vi "Simple_ManualSyringeControl_VB_20170921_synchronousflush.vi"() -> ()   [LabVIEW 2013]
uses:
  <vilib>/Instr/_visa.llb/VISA Configure Serial Port (Instr).vi
  <vilib>/Instr/_visa.llb/VISA Flush IO Buffer Mask.ctl
panel:
  out "Syringe Diameter (mm)":string
  in  "Mask":T1=16 items=["Flush Receive Buffer"=16, "Write Transmit Buffer to Device"=32, "Flush Receive Buffer (No I/O)"=64, "Flush Transmit Buffer"=128]
  out "Pump #":dbl caption="Pumps:" format="%#g"
  out "Sync":bool
  in  "STOP ALL":bool
  in  "RUN ALL":bool
  in  "Synchronous Pumps (T/F)":bool
  in  "Flush Rate (mL/hour)":string="20"
  out "Flushing?":bool
  in  "Flush":bool
  in  "Infuse Rate (mL/hour)":string="2"
  in  "STOP PUMP 01":bool
  in  "RUN PUMP 01":bool
  in  "Mask Init 2":T1=16 items=["Flush Receive Buffer"=16, "Write Transmit Buffer to Device"=32, "Flush Receive Buffer (No I/O)"=64, "Flush Transmit Buffer"=128]
  in  "stop bits (2 bit)":u16(ring)=20 items=["1.0"=10, "1.5"=15, "2.0"=20]
  in  "termination char\n(0xD = '\\r' = CR)":u8=13 format="%.0x"
  in  "data bits (8)":u16=8 min=5 max=8 step=1
  in  "baud rate (9600)":u32=9600
  in  "VISA resource name":refnum<visa-resource-name>="COM3"
  in  "STOP PUMP 00":bool
  in  "Mask Exit":T1=16 items=["Flush Receive Buffer"=16, "Write Transmit Buffer to Device"=32, "Flush Receive Buffer (No I/O)"=64, "Flush Transmit Buffer"=128]
  in  "RUN PUMP 00":bool
  in  "Mask Initialize 2":T1=16 items=["Flush Receive Buffer"=16, "Write Transmit Buffer to Device"=32, "Flush Receive Buffer (No I/O)"=64, "Flush Transmit Buffer"=128]
  in  "Mask Init":T1=16 items=["Flush Receive Buffer"=16, "Write Transmit Buffer to Device"=32, "Flush Receive Buffer (No I/O)"=64, "Flush Transmit Buffer"=128]
  out "Response":string
  out "Response Blank":string
  in  "Command:":string
  in  "Pump Address":enum16{"00", "01", "02", "03"}(ring)
  in  "OK Button":bool
  in  "EXIT PROGRAM":bool
  # "UPON START-UP: User is asked to input number of pumps being used and diameter of syringe"
  # "DURING RUN: Default Infusion Rate is 2 mL/hour, to change this, modify Infusion Rate before giving RUN command or pressing PLAY"
  # "OFF"
  # "ON"
  # "COMMANDS LIST\n\nRUN Start infuse (forward direction)\nRUNW Starts withdraw (reverse direction)\nSTP Stop motor\nCLV Clears infuse volume accumulator to zero\nCLT Clears target infuse volume to zero, dispense disabled\nCLTW Clears target withdraw volume to zero\nMAX Sets the pump to the maximum infuse flow rate\n\nCommands with Numbers \n(Number Range: 0-1999)\n(Must have space before number)\nFOR Force setting as percentage (number can be 0-100).\nMLH Set infuse flow rate and range, units are milliliters per hour.\nULT  Set target infusion volume, units are µl .\nMLT Set target infusion volume, units are ml.\n\nSee Harvard Apparatus OEM Millimeter pump manual for more commands and details."
  # "QUERIES LIST \n\nDIA Returns diameter value units in mm\nRAT Returns infusion rate value set in current range units\nRATW Returns withdraw rate value set in current range units\nVOL Returns current accumulated infused volume, units in ml or µl\ndepending on range.\nVOLW Returns current accumulated withdraw volume, units in ml or µl\ndepending on range.\nVER Returns model and version number of firmware\nTAR Returns target infuse volume, units in ml or µl depending on range \nFRC Returns force setting and percent\nRNG Returns infuse range message (character string either: ML/H, ML/M,\nUL/H, UL/M)\nEMG Returns emergency stop input status (True/False); True =\nEmergency Stop\nLIM Returns “*I”, “*W” or “false”; indicating limit switch actuation status."
  # "Individual Control"
  # ": stopped\n> running forward\n*I stalled"
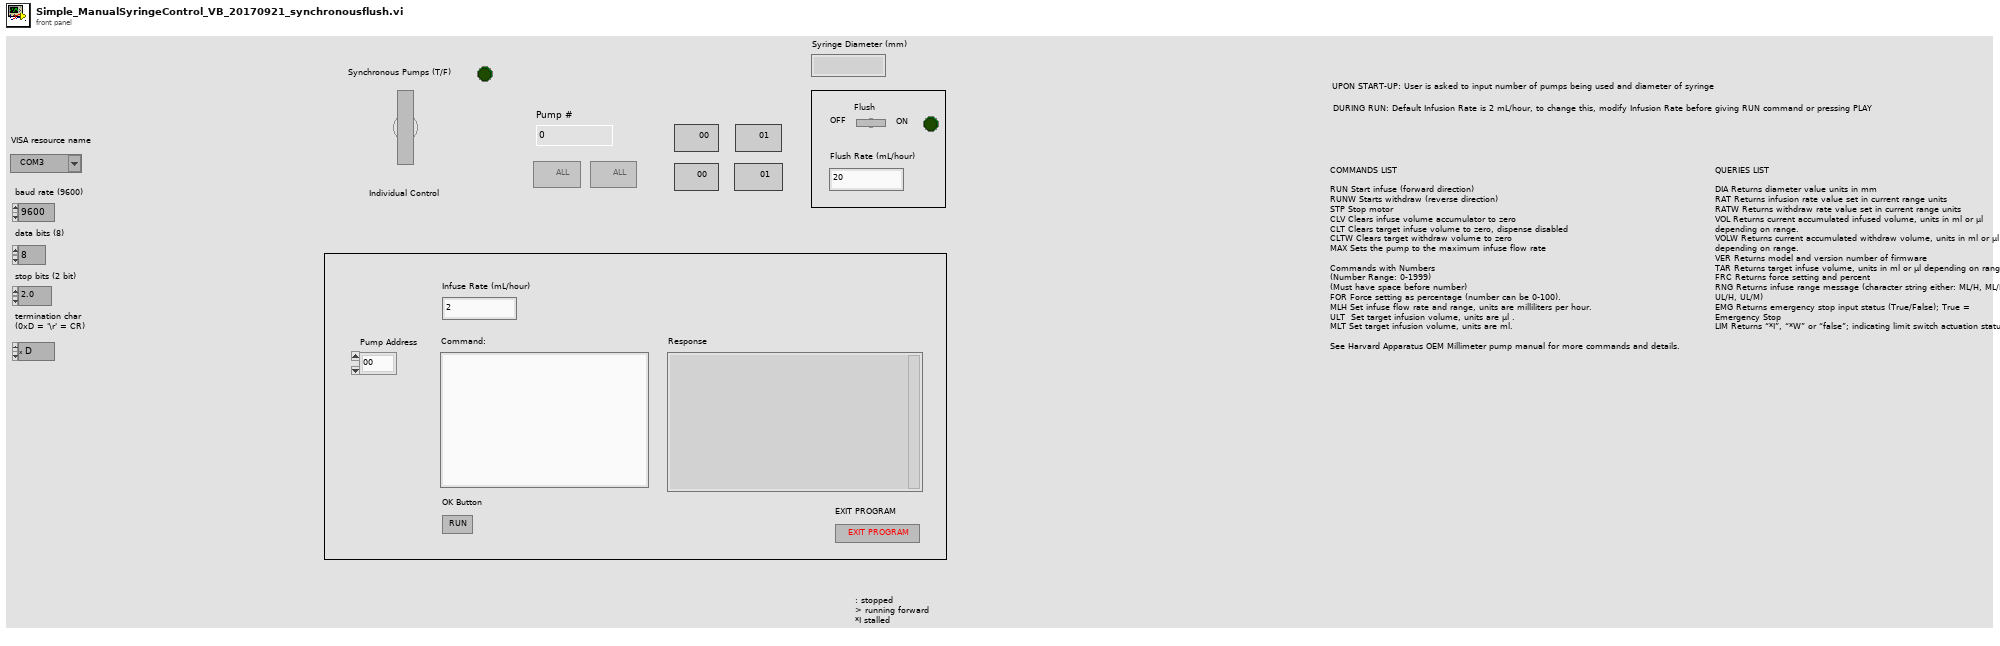
[diagram p1: front panel]
types:
  T1 = typedef "VISA Flush IO Buffer Mask.ctl" = u16
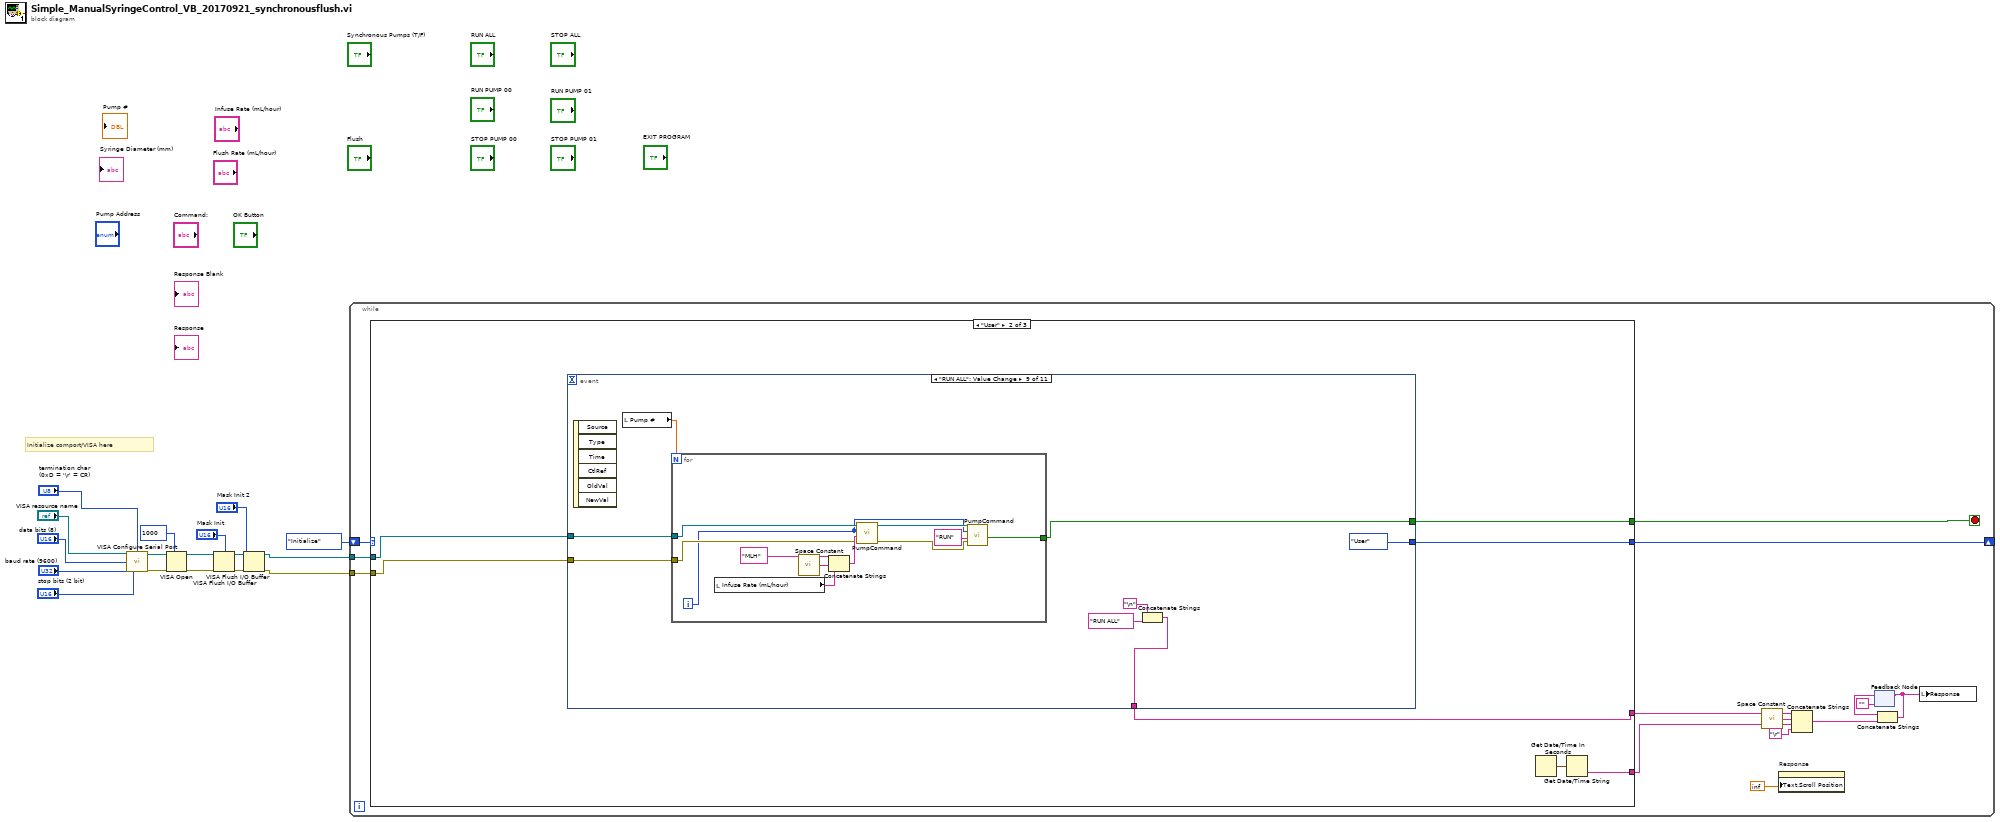
[diagram p0: block diagram]
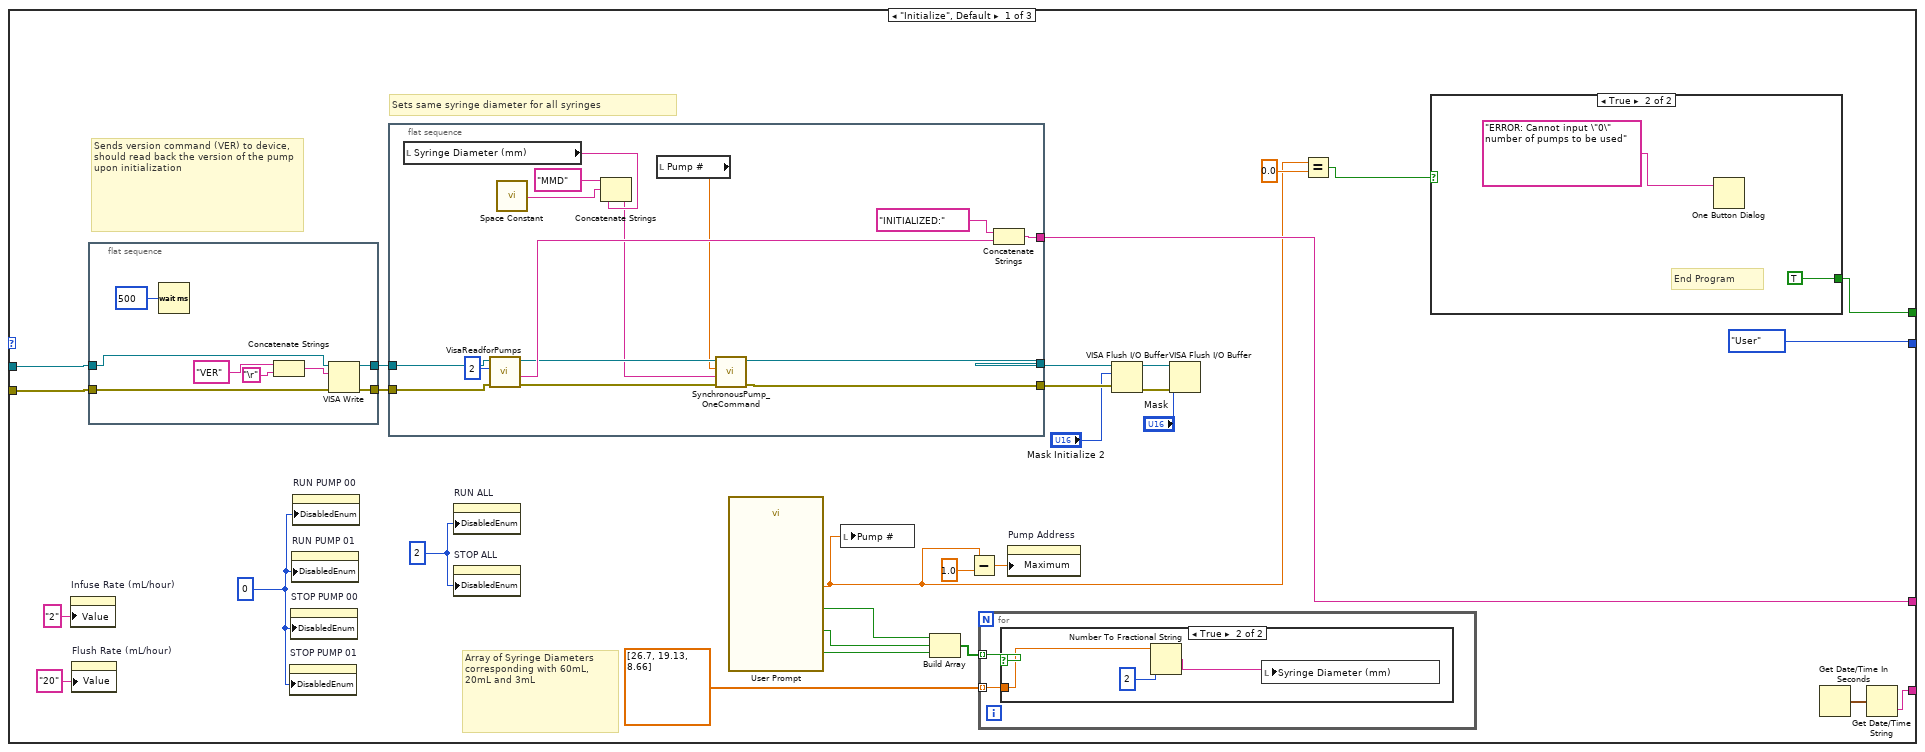
[diagram p2: hidden frame]
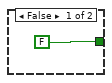
[diagram p3: hidden frame]
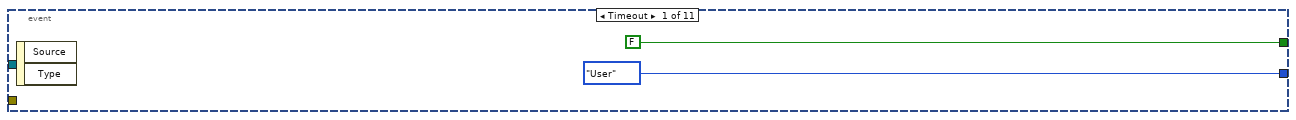
[diagram p5: hidden frame]
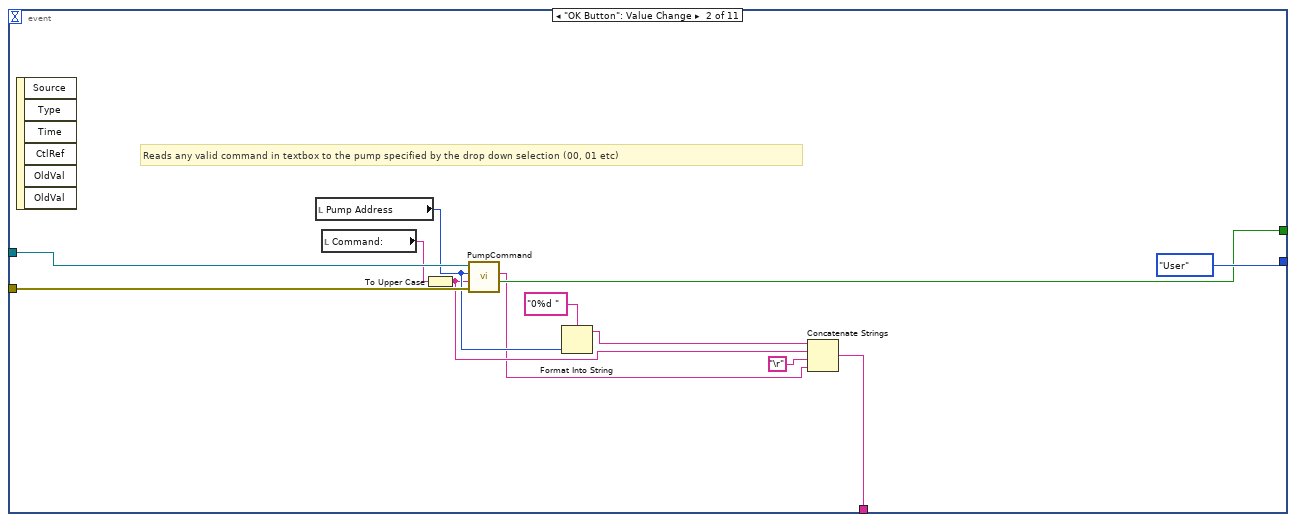
[diagram p6: hidden frame]
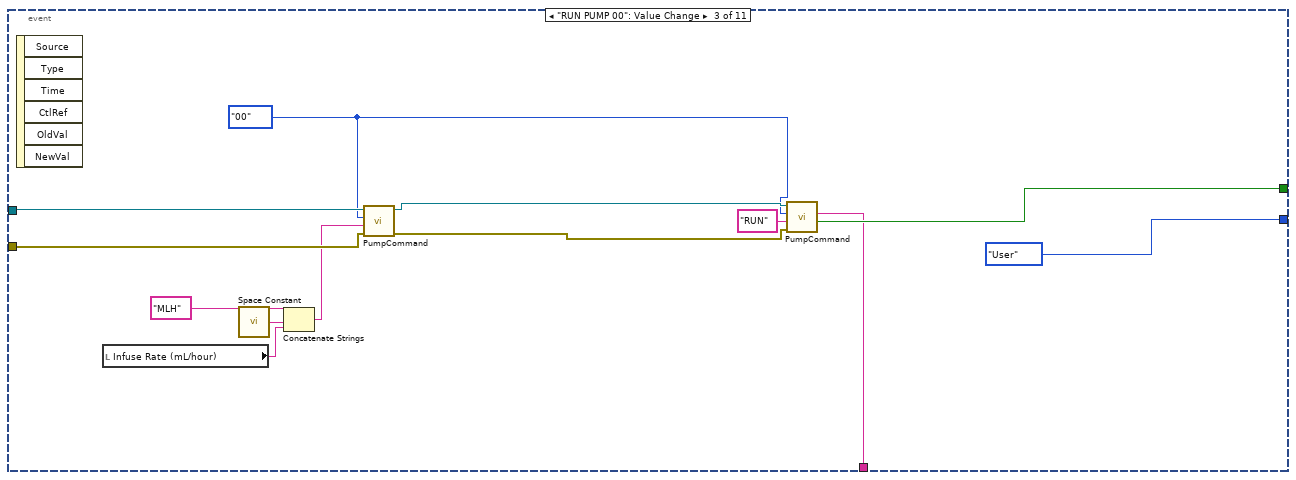
[diagram p7: hidden frame]
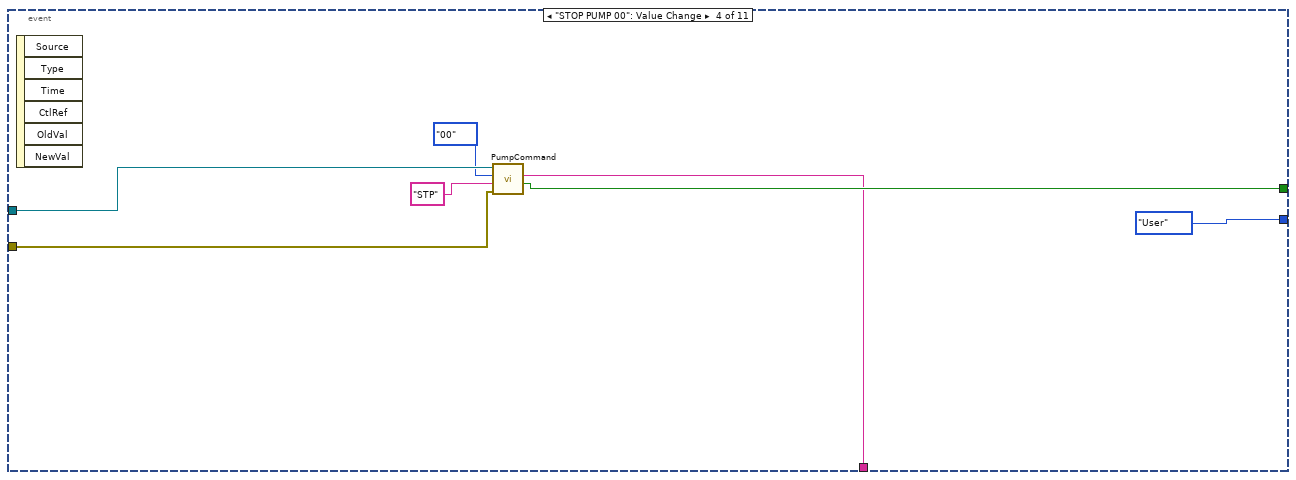
[diagram p8: hidden frame]
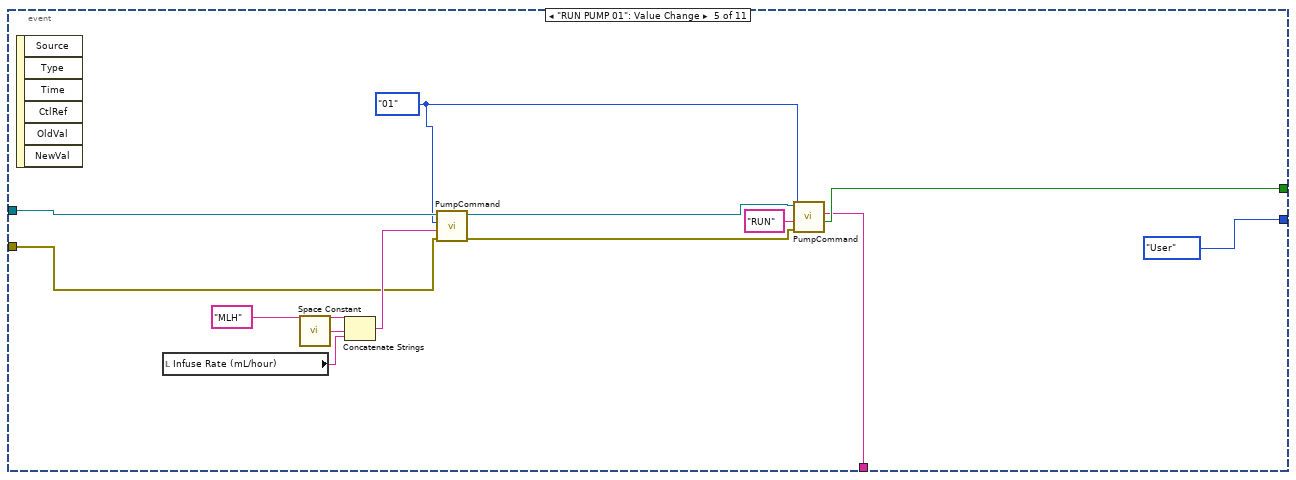
[diagram p9: hidden frame]
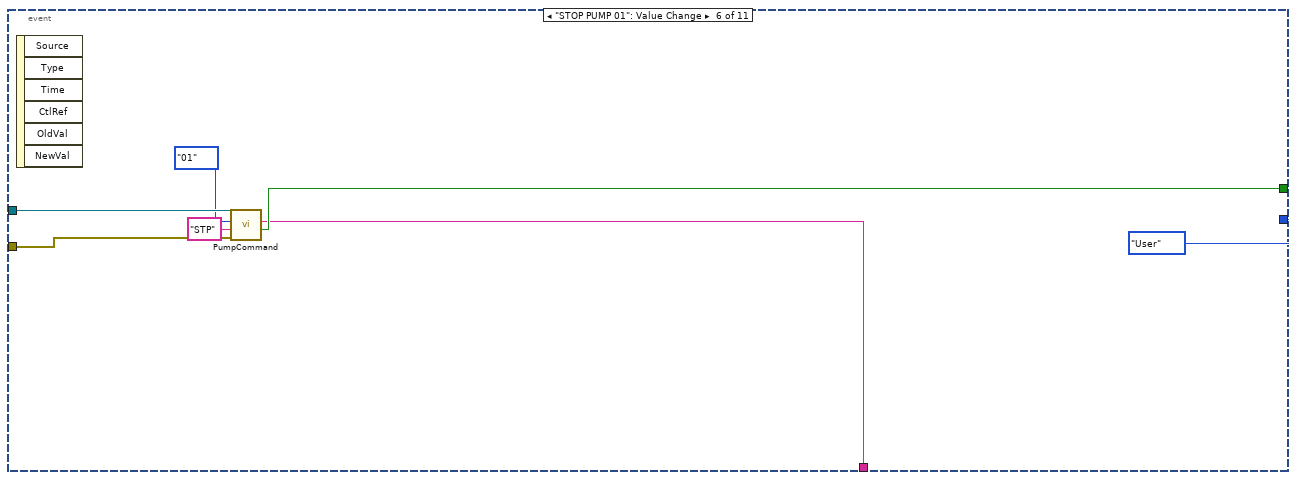
[diagram p10: hidden frame]
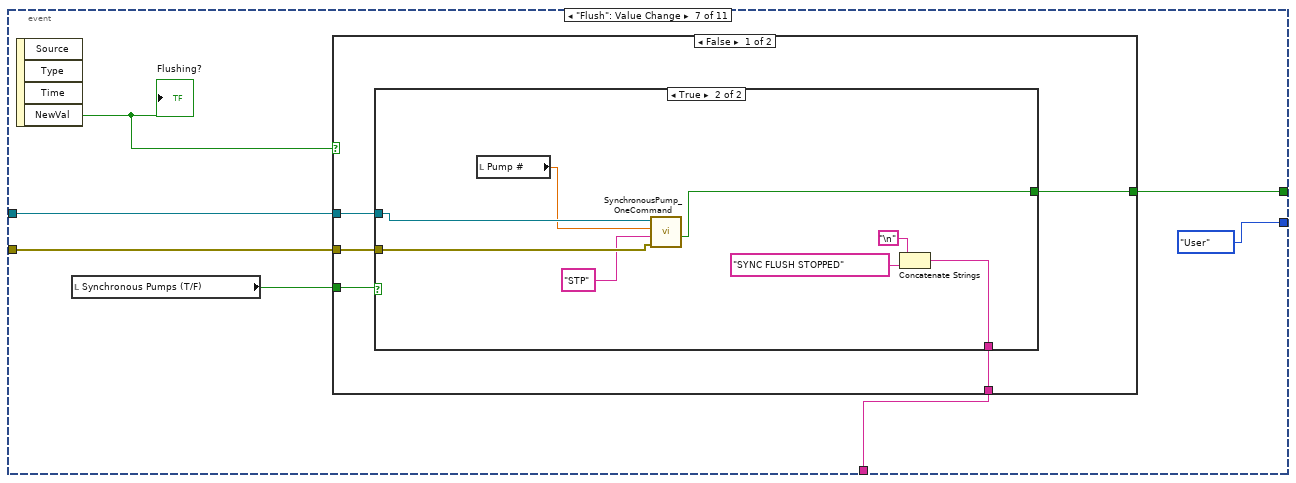
[diagram p11: hidden frame]
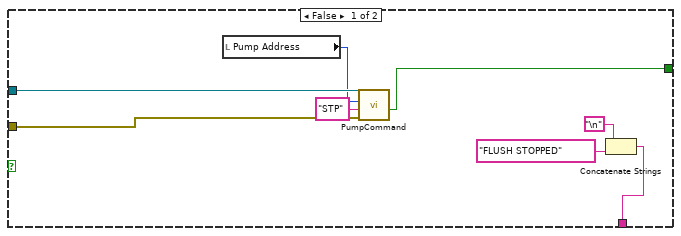
[diagram p12: hidden frame]
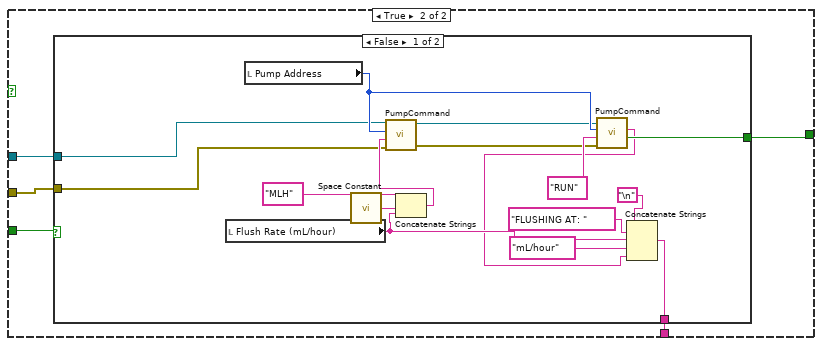
[diagram p13: hidden frame]
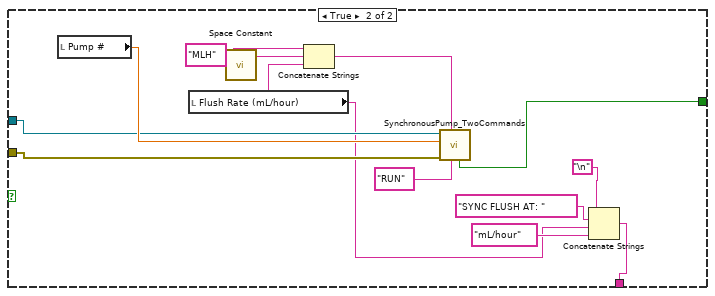
[diagram p14: hidden frame]
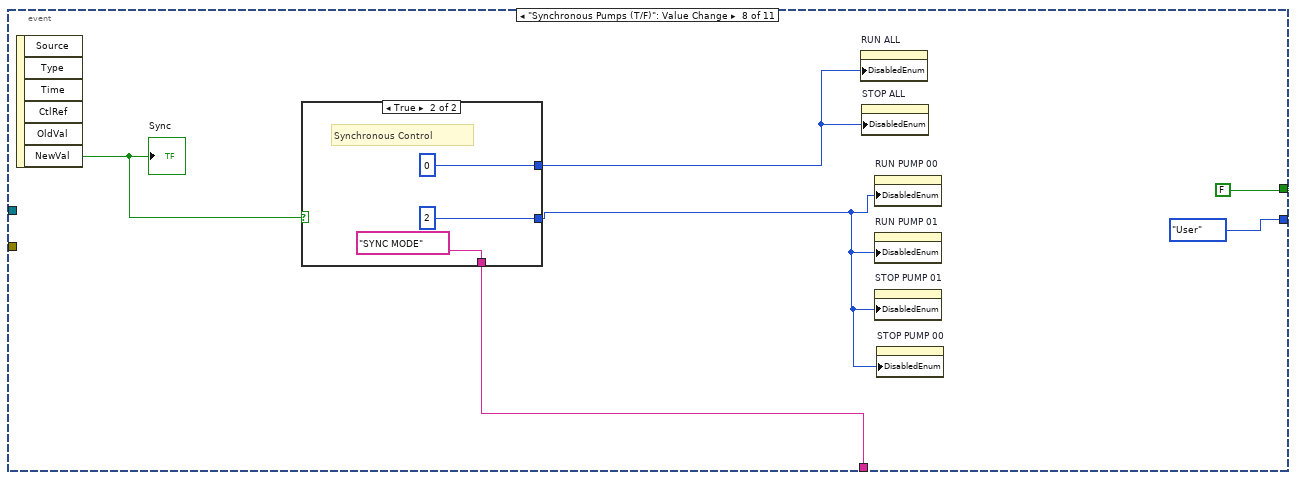
[diagram p15: hidden frame]
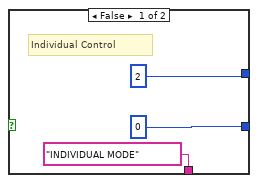
[diagram p16: hidden frame]
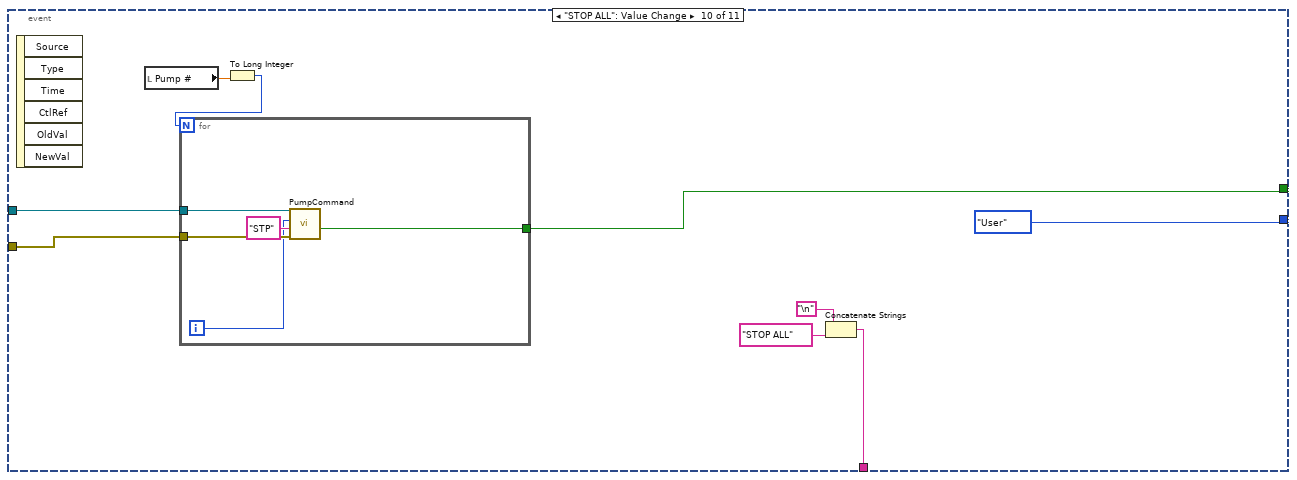
[diagram p17: hidden frame]
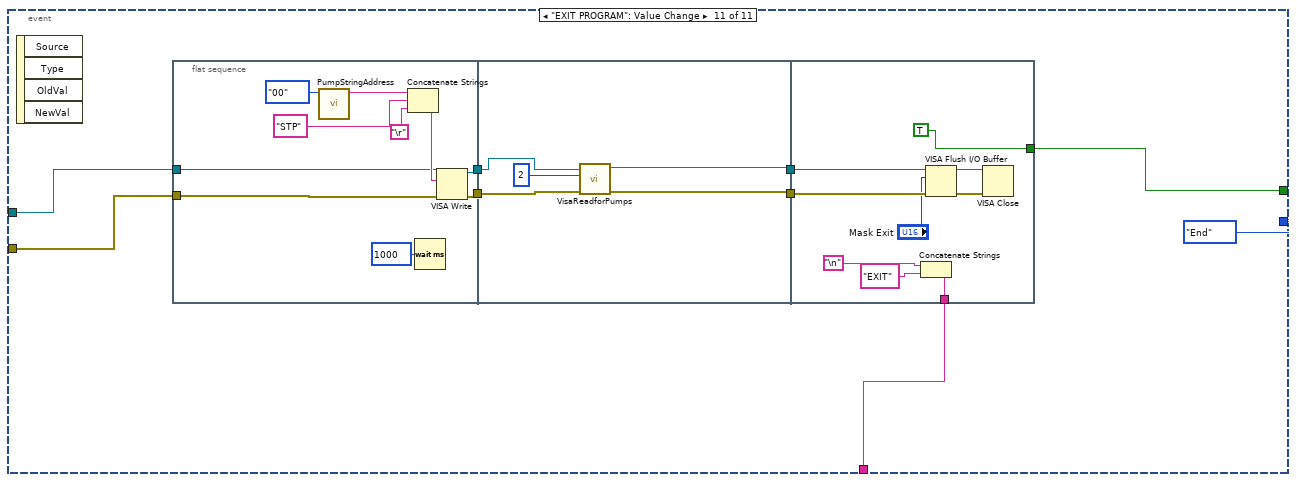
[diagram p18: hidden frame]
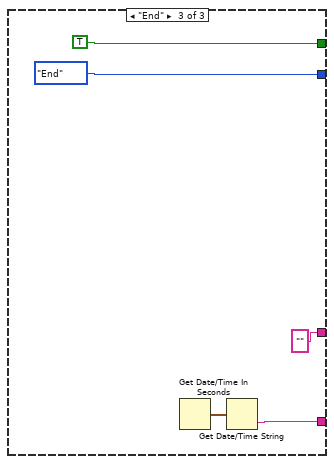
[diagram p19: hidden frame]
diagram:
  # "Initialize comport/VISA here"
  n1 = call-poly "VISA Configure Serial Port"("VISA resource name"="VISA resource name", "termination char\n(0xA = '\\n' = LF)"="termination char\n(0xD = '\\r' = CR)", "baud rate (9600)"="baud rate (9600)", "data bits (8)"="data bits (8)", "stop bits (10: 1 bit)"="stop bits (2 bit)") -> ("VISA resource name out"=w13:refnum<visa-resource-name>, "error out"=w12:errorcluster)  [unwired: 9 in]
  n2 = VISA Open(timeout (0)=1000, error in (no error)=w12, VISA resource name=w13) -> (VISA resource name=w15:refnum<visa-resource-name>, error out=w16:errorcluster)  [unwired: 2 in]
  n3 = VISA Flush I/O Buffer(VISA resource name=w15, mask (16)="Mask Init", error in (no error)=w16) -> (VISA resource name out=w4:refnum<visa-resource-name>, error out=w5:errorcluster)
  n4 = VISA Flush I/O Buffer(VISA resource name=w4, mask (16)="Mask Init 2", error in (no error)=w5) -> (VISA resource name out=w3:refnum<visa-resource-name>, error out=w2:errorcluster)
  n5 = while {
    shift-right: [w30] -> _
    shift-left: enum16{"Initialize", "User", "End"}."Initialize" -> [w29]
    tunnel: w3 -> [w28]
    tunnel: w2 -> [w27]
    stop <- w31 stop-if-true
    n6 = case shown="\"User\"" w29 {
      tunnel: [w33 w97 TRUE] -> w31
      tunnel: [enum16{"Initialize", "User", "End"}."User" w98 enum16{"Initialize", "User", "End"}."End"] -> w30
      tunnel: w28 -> [w55 w96 _]
      tunnel: w27 -> [w54 w95 _]
      tunnel: [w48 w94 "" ("Read (Response)")] -> w21
      tunnel: [w36 w92 w293] -> w18
      frame "Initialize", Default {
        w51 = 2
        w52 = 0
        # "Array of Syringe Diameters corresponding with 60mL, 20mL and 3mL"
        # "Sets same syringe diameter for all syringes"
        # "Sends version command (VER) to device, should read back the version of the pump upon initialization"
        n7 = property on="Infuse Rate (mL/hour)" class="Str"("Value"="2" ("Infuse Rate (mL/hour)")) -> ()  [unwired: 2 in, 2 out]
        n8 = property on="Flush Rate (mL/hour)" class="Str"("Value"="20" ("Flush Rate (mL/hour)")) -> ()  [unwired: 2 in, 2 out]
        n9 = flat-sequence {
          tunnel: [w89] -> w60
          tunnel: [w88] -> w59
          tunnel: w55 -> [w86]
          tunnel: w54 -> [w85]
          frame #0 {
            n10 = Wait (ms)(milliseconds to wait=500) -> ()  [unwired: 1 out]
            n11 = Concatenate Strings("VER", "\r") -> (w90:string)
            n12 = VISA Write(VISA resource name=w86, write buffer=w90, error in (no error)=w85) -> (VISA resource name out=w89:refnum<visa-resource-name>, error out=w88:errorcluster)  [unwired: 1 out]
          }
        }
        n13 = property on="STOP PUMP 01" class="Bool"("DisabledEnum"=w52) -> ()  [unwired: 2 in, 2 out]
        n14 = property on="STOP PUMP 00" class="Bool"("DisabledEnum"=w52) -> ()  [unwired: 2 in, 2 out]
        n15 = property on="RUN PUMP 01" class="Bool"("DisabledEnum"=w52) -> ()  [unwired: 2 in, 2 out]
        n16 = property on="RUN PUMP 00" class="Bool"("DisabledEnum"=w52) -> ()  [unwired: 2 in, 2 out]
        n17 = flat-sequence {
          tunnel: w60 -> [w81]
          tunnel: w59 -> [w80]
          tunnel: [w76] -> w57
          tunnel: [w75] -> w56
          tunnel: [w82] -> w48
          frame #0 {
            n18 = local read "Syringe Diameter (mm)"() -> (w71:string)
            n19 = call "VisaReadforPumps.vi"("error in (no error)"=w80, "Byte Count"=2, "VISA Refnum in"=w81) -> ("error out"=w77:errorcluster, "Read (Response)"=w79:string, "VISA Refnum out"=w78:refnum<visa-resource-name>)  [unwired: 5 in, 1 out]
            n20 = call <vilib>:"Space Constant.vi"() -> ("String"=w72:string)
            n21 = Concatenate Strings("MMD" ("Command:"), w72, w71) -> (w69:string)
            n22 = local read "Pump #"() -> (w70:dbl)
            n23 = call "SynchronousPump_OneCommand.vi"("error in (no error)"=w77, "Command"=w69, "Pump #"=w70, "VISA Refnum in"=w78) -> ("error out"=w75:errorcluster, "VISA Refnum out"=w76:refnum<visa-resource-name>)  [unwired: 4 in, 2 out]
            n24 = Concatenate Strings("INITIALIZED:", w79) -> (w82:string)
          }
        }
        n25 = property on="RUN ALL" class="Bool"("DisabledEnum"=w51) -> ()  [unwired: 2 in, 2 out]
        n26 = property on="STOP ALL" class="Bool"("DisabledEnum"=w51) -> ()  [unwired: 2 in, 2 out]
        n27 = call "User Prompt"() -> ("BD, 3 mL"=w42:bool, "BD, 20 mL"=w43:bool, "BD, 60 mL"=w44:bool, "Pumps:"=w32:dbl)  [unwired: 14 in, 2 out]
        n28 = local write "Pump #"(w32) -> ()
        n29 = Build Array(w44, w43, w42) -> (w41:bool[])
        n30 = Subtract(x=w32, y=1.0) -> (x-y=w50:dbl)
        n31 = for {
          tunnel: w41 -> [w65] mode=indexing
          tunnel: dbl[] [26.7, 19.13, 8.66] -> [w64] mode=indexing
          n32 = case shown="True" w65 {
            tunnel: w64 -> [_ w66]
            frame False {
            }
            frame True {
              n33 = Number To Fractional String(number=w66, precision (6)=i16 2) -> (F-format string=w68:string)  [unwired: 2 in]
              n34 = local write "Syringe Diameter (mm)"(w68) -> ()
            }
          }
        }
        n35 = property on="Pump Address" class="Enum (strict)"("Maximum"=w50) -> ()  [unwired: 2 in, 2 out]
        n36 = VISA Flush I/O Buffer(VISA resource name=w57, mask (16)="Mask Initialize 2", error in (no error)=w56) -> (VISA resource name out=w47:refnum<visa-resource-name>, error out=w46:errorcluster)
        n37 = VISA Flush I/O Buffer(VISA resource name=w47, mask (16)="Mask", error in (no error)=w46) -> ()  [unwired: 2 out]
        n38 = Equal?(x=w32, y=0.0) -> (x = y?=w34:bool)
        n39 = case shown="True" w34 {
          tunnel: [FALSE TRUE] -> w33
          frame False {
          }
          frame True {
            # "End Program"
            n40 = One Button Dialog(message="ERROR: Cannot input \"0\" number of pumps to be used") -> ()  [unwired: 1 in, 1 out]
          }
        }
        n41 = Get Date/Time In Seconds() -> (seconds since 1Jan1904=w37:timestamp)
        n42 = Get Date/Time String(seconds (now)=w37) -> (time string=w36:string)  [unwired: 2 in, 1 out]
      }
      frame "User" {
        n43 = event shown="[8] \"RUN ALL\": Value Change" {
          selector: _ -> [_ _ _ _ _ _ _ _ _ _ _]
          dyn-events: _ -> [_ _ _ _ _ _ _ _ _ _ _]
          timeout: _ -> [_ _ _ _ _ _ _ _ _ _ _]
          tunnel: [enum16{"Initialize", "User", "End"}."User" enum16{"Initialize", "User", "End"}."User" enum16{"Initialize", "User", "End"}."User" enum16{"Initialize", "User", "End"}."User" enum16{"Initialize", "User", "End"}."User" enum16{"Initialize", "User", "End"}."User" enum16{"Initialize", "User", "End"}."User" enum16{"Initialize", "User", "End"}."User" enum16{"Initialize", "User", "End"}."User" enum16{"Initialize", "User", "End"}."User" enum16{"Initialize", "User", "End"}."End"] -> w98
          tunnel: [FALSE w109 w124 w129 w144 w148 w156 FALSE w230 w249 w267] -> w97
          tunnel: w96 -> [_ w111 w120 w131 w137 w152 w158 _ w233 w254 w262]
          tunnel: w95 -> [_ w110 w119 w132 w136 w151 w157 _ w232 w253 w261]
          tunnel: [_ w103 w113 w126 w133 w146 w154 w215 w228 w247 w260] -> w94
          event Timeout {
            n44 = event-data() -> ()  [unwired: 1 in, 2 out]
          }
          event "OK Button": Value Change {
            # "Reads any valid command in textbox to the pump specified by the drop down selection (00, 01 etc)"
            n45 = event-data() -> ()  [unwired: 1 in, 6 out]
            n46 = local read "Pump Address"() -> (w107:enum16{"00", "01", "02", "03"})
            n47 = local read "Command:"() -> (w108:string)
            n48 = To Upper Case(1:w108) -> (0:w104:string)
            n49 = call "PumpCommand.vi"("error in (no error)"=w110, "Command:"=w104, "Pump Address"=w107, "VISA Refnum in"=w111) -> ("EXIT PROGRAM? (F)"=w109:bool, "Read (Response)"=w102:string)  [unwired: 3 in, 2 out]
            n50 = Format Into String(format string="0%d ", w107) -> (resulting string=w105:string)  [unwired: 2 in, 1 out]
            n51 = Concatenate Strings(w105, w104, "\r", w102) -> (w103:string)
          }
          event "RUN PUMP 00": Value Change {
            w118 = enum16{"00", "01", "02", "03"}."00" ("Pump Address")
            n52 = event-data() -> ()  [unwired: 1 in, 6 out]
            n53 = local read "Infuse Rate (mL/hour)"() -> (w116:string)
            n54 = call <vilib>:"Space Constant.vi"() -> ("String"=w115:string)
            n55 = Concatenate Strings("MLH" ("Command:"), w115, w116) -> (w114:string)
            n56 = call "PumpCommand.vi"("error in (no error)"=w119, "Command:"=w114, "Pump Address"=w118, "VISA Refnum in"=w120) -> ("error out"=w121:errorcluster, "VISA resource name out"=w122:refnum<visa-resource-name>)  [unwired: 3 in, 2 out]
            n57 = call "PumpCommand.vi"("error in (no error)"=w121, "Command:"="RUN", "Pump Address"=w118, "VISA Refnum in"=w122) -> ("EXIT PROGRAM? (F)"=w124:bool, "Read (Response)"=w113:string)  [unwired: 3 in, 2 out]
          }
          event "STOP PUMP 00": Value Change {
            n58 = event-data() -> ()  [unwired: 1 in, 6 out]
            n59 = call "PumpCommand.vi"("error in (no error)"=w132, "Command:"="STP", "Pump Address"=enum16{"00", "01", "02", "03"}."00", "VISA Refnum in"=w131) -> ("EXIT PROGRAM? (F)"=w129:bool, "Read (Response)"=w126:string)  [unwired: 3 in, 2 out]
          }
          event "RUN PUMP 01": Value Change {
            w134 = enum16{"00", "01", "02", "03"}."01" ("Pump Address")
            n60 = event-data() -> ()  [unwired: 1 in, 6 out]
            n61 = local read "Infuse Rate (mL/hour)"() -> (w135:string)
            n62 = call <vilib>:"Space Constant.vi"() -> ("String"=w141:string)
            n63 = Concatenate Strings("MLH" ("Command:"), w141, w135) -> (w140:string)
            n64 = call "PumpCommand.vi"("error in (no error)"=w136, "Command:"=w140, "Pump Address"=w134, "VISA Refnum in"=w137) -> ("error out"=w138:errorcluster, "VISA resource name out"=w139:refnum<visa-resource-name>)  [unwired: 3 in, 2 out]
            n65 = call "PumpCommand.vi"("error in (no error)"=w138, "Command:"="RUN", "Pump Address"=w134, "VISA Refnum in"=w139) -> ("EXIT PROGRAM? (F)"=w144:bool, "Read (Response)"=w133:string)  [unwired: 3 in, 2 out]
          }
          event "STOP PUMP 01": Value Change {
            n66 = event-data() -> ()  [unwired: 1 in, 6 out]
            n67 = call "PumpCommand.vi"("error in (no error)"=w151, "Command:"="STP", "Pump Address"=enum16{"00", "01", "02", "03"}."01", "VISA Refnum in"=w152) -> ("EXIT PROGRAM? (F)"=w148:bool, "Read (Response)"=w146:string)  [unwired: 3 in, 2 out]
          }
          event "Flush": Value Change {
            n68 = event-data() -> ("NewVal"=w159:bool)  [unwired: 1 in, 3 out]
            "Flushing?" <- w159
            n69 = local read "Synchronous Pumps (T/F)"() -> (w153:bool)
            n70 = case shown="False" w159 {
              tunnel: w158 -> [w164 w185]
              tunnel: w157 -> [w163 w184]
              tunnel: [w162 w183] -> w156
              tunnel: [w161 w182] -> w154
              tunnel: w153 -> [w160 w181]
              frame False {
                n71 = case shown="True" w160 {
                  tunnel: w164 -> [w172 w180]
                  tunnel: w163 -> [w171 w179]
                  tunnel: [w168 w177] -> w162
                  tunnel: [w166 w174] -> w161
                  frame False {
                    n72 = local read "Pump Address"() -> (w170:enum16{"00", "01", "02", "03"})
                    n73 = call "PumpCommand.vi"("error in (no error)"=w171, "Command:"="STP", "Pump Address"=w170, "VISA Refnum in"=w172) -> ("EXIT PROGRAM? (F)"=w168:bool)  [unwired: 3 in, 3 out]
                    n74 = Concatenate Strings("\n", "FLUSH STOPPED") -> (w166:string)
                  }
                  frame True {
                    n75 = local read "Pump #"() -> (w173:dbl)
                    n76 = call "SynchronousPump_OneCommand.vi"("error in (no error)"=w179, "Command"="STP", "Pump #"=w173, "VISA Refnum in"=w180) -> ("EXIT PROGRAM? (F)"=w177:bool)  [unwired: 4 in, 3 out]
                    n77 = Concatenate Strings("\n", "SYNC FLUSH STOPPED") -> (w174:string)
                  }
                }
              }
              frame True {
                n78 = case shown="False" w181 {
                  tunnel: w185 -> [w194 w213]
                  tunnel: w184 -> [w193 w212]
                  tunnel: [w192 w209] -> w183
                  tunnel: [w188 w204] -> w182
                  frame False {
                    n79 = local read "Flush Rate (mL/hour)"() -> (w189:string)
                    n80 = local read "Pump Address"() -> (w200:enum16{"00", "01", "02", "03"})
                    n81 = call <vilib>:"Space Constant.vi"() -> ("String"=w195:string)
                    n82 = Concatenate Strings("MLH" ("Command:"), w195, w189) -> (w197:string)
                    n83 = call "PumpCommand.vi"("error in (no error)"=w193, "Command:"=w197, "Pump Address"=w200, "VISA Refnum in"=w194) -> ("error out"=w199:errorcluster, "VISA resource name out"=w198:refnum<visa-resource-name>)  [unwired: 3 in, 2 out]
                    n84 = call "PumpCommand.vi"("error in (no error)"=w199, "Command:"="RUN", "Pump Address"=w200, "VISA Refnum in"=w198) -> ("EXIT PROGRAM? (F)"=w192:bool, "Read (Response)"=w186:string)  [unwired: 3 in, 2 out]
                    n85 = Concatenate Strings("\n", "FLUSHING AT: " ("string"), w189, "mL/hour" ("string"), w186) -> (w188:string)
                  }
                  frame True {
                    n86 = local read "Pump #"() -> (w214:dbl)
                    n87 = local read "Flush Rate (mL/hour)"() -> (w203:string)
                    n88 = call <vilib>:"Space Constant.vi"() -> ("String"=w211:string)
                    n89 = Concatenate Strings("MLH" ("Command:"), w211, w203) -> (w208:string)
                    n90 = call "SynchronousPump_TwoCommands.vi"("Command 2"="RUN", "Command 1"=w208, "error in (no error)"=w212, "Pump #"=w214, "VISA Refnum in"=w213) -> ("EXIT PROGRAM? (F)"=w209:bool)  [unwired: 2 in, 4 out]
                    n91 = Concatenate Strings("\n", "SYNC FLUSH AT: " ("string"), w203, "mL/hour" ("string")) -> (w204:string)
                  }
                }
              }
            }
          }
          event "Synchronous Pumps (T/F)": Value Change {
            n92 = event-data() -> ("NewVal"=w220:bool)  [unwired: 1 in, 5 out]
            "Sync" <- w220
            n93 = case shown="True" w220 {
              tunnel: [0 2] -> w219
              tunnel: [2 0] -> w218
              tunnel: ["INDIVIDUAL MODE" "SYNC MODE"] -> w215
              frame False {
                # "Individual Control"
              }
              frame True {
                # "Synchronous Control"
              }
            }
            n94 = property on="RUN ALL" class="Bool"("DisabledEnum"=w218) -> ()  [unwired: 2 in, 2 out]
            n95 = property on="STOP ALL" class="Bool"("DisabledEnum"=w218) -> ()  [unwired: 2 in, 2 out]
            n96 = property on="RUN PUMP 00" class="Bool"("DisabledEnum"=w219) -> ()  [unwired: 2 in, 2 out]
            n97 = property on="RUN PUMP 01" class="Bool"("DisabledEnum"=w219) -> ()  [unwired: 2 in, 2 out]
            n98 = property on="STOP PUMP 01" class="Bool"("DisabledEnum"=w219) -> ()  [unwired: 2 in, 2 out]
            n99 = property on="STOP PUMP 00" class="Bool"("DisabledEnum"=w219) -> ()  [unwired: 2 in, 2 out]
          }
          event "RUN ALL": Value Change {
            n100 = event-data() -> ()  [unwired: 1 in, 6 out]
            n101 = local read "Pump #"() -> (w231:dbl)
            n102 = for {
              N: w231 -> [_]
              tunnel: w233 -> [w238]
              tunnel: w232 -> [w237]
              tunnel: [w235] -> w230
              i -> [w236]
              n103 = local read "Infuse Rate (mL/hour)"() -> (w239:string)
              n104 = call <vilib>:"Space Constant.vi"() -> ("String"=w242:string)
              n105 = Concatenate Strings("MLH" ("Command:"), w242, w239) -> (w240:string)
              n106 = call "PumpCommand.vi"("error in (no error)"=w237, "Command:"=w240, "Pump Address"=w236, "VISA Refnum in"=w238) -> ("error out"=w243:errorcluster, "VISA resource name out"=w244:refnum<visa-resource-name>)  [unwired: 3 in, 2 out]
              n107 = call "PumpCommand.vi"("error in (no error)"=w243, "Command:"="RUN", "Pump Address"=w236, "VISA Refnum in"=w244) -> ("EXIT PROGRAM? (F)"=w235:bool)  [unwired: 3 in, 3 out]
            }
            n108 = Concatenate Strings("\n", "RUN ALL" ("Read (Response)")) -> (w228:string)
          }
          event "STOP ALL": Value Change {
            n109 = event-data() -> ()  [unwired: 1 in, 6 out]
            n110 = local read "Pump #"() -> (w252:dbl)
            n111 = To Long Integer(number=w252) -> (32bit integer=w251:i32)
            n112 = for {
              N: w251 -> [_]
              tunnel: w254 -> [w259]
              tunnel: w253 -> [w258]
              tunnel: [w255] -> w249
              i -> [w256]
              n113 = call "PumpCommand.vi"("error in (no error)"=w258, "Command:"="STP", "Pump Address"=w256, "VISA Refnum in"=w259) -> ("EXIT PROGRAM? (F)"=w255:bool)  [unwired: 3 in, 3 out]
            }
            n114 = Concatenate Strings("\n", "STOP ALL" ("Read (Response)")) -> (w247:string)
          }
          event "EXIT PROGRAM": Value Change {
            n115 = event-data() -> ()  [unwired: 1 in, 4 out]
            n116 = flat-sequence {
              tunnel: [w277] -> w266
              tunnel: [w276] -> w265
              tunnel: w262 -> [w272]
              tunnel: w261 -> [w271]
              tunnel: w266 -> [w283]
              tunnel: w265 -> [w281]
              tunnel: [w280] -> w264
              tunnel: [w279] -> w263
              tunnel: [TRUE] -> w267
              tunnel: w264 -> [w289]
              tunnel: w263 -> [w288]
              tunnel: [w286] -> w260
              frame #0 {
                n117 = call "PumpStringAddress.vi"("Pump Address"=enum16{"00", "01", "02", "03"}."00") -> ("String"=w275:string)  [unwired: 10 in]
                n118 = Concatenate Strings(w275, "STP", "\r") -> (w278:string)
                n119 = Wait (ms)(milliseconds to wait=1000) -> ()  [unwired: 1 out]
                n120 = VISA Write(VISA resource name=w272, write buffer=w278, error in (no error)=w271) -> (VISA resource name out=w277:refnum<visa-resource-name>, error out=w276:errorcluster)  [unwired: 1 out]
              }
              frame #1 {
                n121 = call "VisaReadforPumps.vi"("error in (no error)"=w281, "Byte Count"=u32 2 ("byte count"), "VISA Refnum in"=w283) -> ("error out"=w279:errorcluster, "VISA Refnum out"=w280:refnum<visa-resource-name>)  [unwired: 5 in, 2 out]
              }
              frame #2 {
                n122 = Concatenate Strings("\n", "EXIT") -> (w286:string)
                n123 = VISA Flush I/O Buffer(VISA resource name=w289, mask (16)="Mask Exit", error in (no error)=w288) -> (VISA resource name out=w290:refnum<visa-resource-name>, error out=w291:errorcluster)
                n124 = VISA Close(VISA resource name=w290, error in (no error)=w291) -> ()  [unwired: 1 out]
              }
            }
          }
        }
        n125 = Get Date/Time In Seconds() -> (seconds since 1Jan1904=w93:timestamp)
        n126 = Get Date/Time String(seconds (now)=w93) -> (time string=w92:string)  [unwired: 2 in, 1 out]
      }
      frame "End" {
        n127 = Get Date/Time In Seconds() -> (seconds since 1Jan1904=w294:timestamp)
        n128 = Get Date/Time String(seconds (now)=w294) -> (time string=w293:string)  [unwired: 2 in, 1 out]
      }
    }
    n129 = call <vilib>:"Space Constant.vi"() -> ("String"=w20:string)
    n130 = property on="Response" class="Str"("Text.Scroll Position"=inf) -> ()  [unwired: 2 in, 2 out]
    n131 = Concatenate Strings(w21, w20, w18, "\r") -> (w22:string)
    n132 = feedback #1("") -> (w26:string)
    n133 = Concatenate Strings(w26, w22) -> (w24:string)
    n134 = feedback-in #1(w24) -> ()
    n135 = local write "Response"(w24) -> ()
  }
